vi "CB Update Model.vi"(9 "u(k)":dbl[](array[numeric]), 10 "x(k)":dbl[](array[numeric]), 11 "State Space Model":T1) -> (2 "y(k+1)":dbl[](array[numeric]) format="%.2f", 3 "x(k+1)":dbl[](array[numeric]) format="%.2f")   [LabVIEW 2020]
uses:
  CB State Space.ctl
  <vilib>/Analysis/Matrix/Datatypes/RealMatrix.ctl
  <vilib>/Analysis/baseanly.llb/A x Vector.vi
  <vilib>/Analysis/NI_AALBase.lvlib
  <vilib>/Analysis/Matrix/NI_Matrix.lvlib
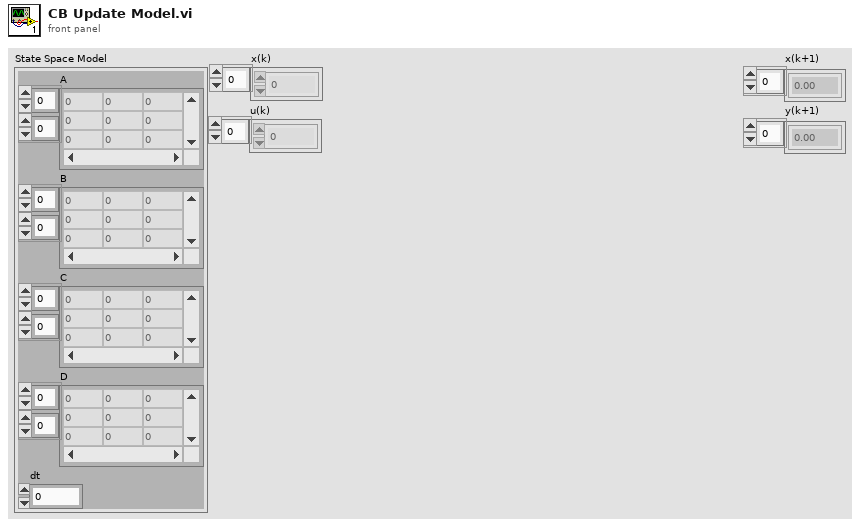
[diagram p1: front panel]
types:
  T1 = typedef "CB State Space.ctl" = cluster{"A":T2, "B":T2, "C":T2, "D":T2, "dt":dbl}
  T2 = typedef "NI_Matrix.lvlib/RealMatrix.ctl" = dbl[][]
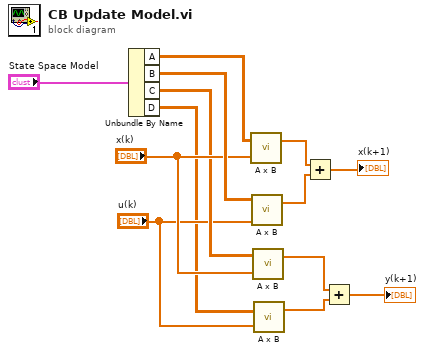
[diagram p0: block diagram]
diagram:
  n1 = Unbundle By Name("State Space Model") -> ("A"=w12:T2, "B"=w11:T2, "C"=w6:T2, "D"=w4:T2)
  n2 = call-poly <vilib>:"A x B.vi"("Vector"="x(k)", "A"=w12) -> ("A x Vector"=w10:dbl[])  [unwired: 1 out]
  n3 = call-poly <vilib>:"A x B.vi"("Vector"="u(k)", "A"=w11) -> ("A x Vector"=w9:dbl[])  [unwired: 1 out]
  n4 = call-poly <vilib>:"A x B.vi"("Vector"="x(k)", "A"=w6) -> ("A x Vector"=w3:dbl[])  [unwired: 1 out]
  n5 = call-poly <vilib>:"A x B.vi"("Vector"="u(k)", "A"=w4) -> ("A x Vector"=w2:dbl[])  [unwired: 1 out]
  n6 = Add(x=w10, y=w9) -> (x+y=→"x(k+1)":dbl[])
  n7 = Add(x=w3, y=w2) -> (x+y=→"y(k+1)":dbl[])
